vi "Read From I16 File.vi"(8 "start of read offset (bytes:0)":i32, 9 "2D number of columns/1D count (all as 1D:-1)":i32=-1, 10 "2D number of rows":i32, 11 "file path (dialog if empty)":path) -> (0 "mark after read (bytes)":i32, 1 "1D array":i16[](array[numeric]), 2 "2D array":i16[][](array[numeric]), 3 "new file path (Not A Path if cancelled)":path, 4 "EOF?":bool)   [LabVIEW 2009]
doc: "Reads a 2D or 1D array of data from a byte stream file of 16-bit signed integers."
panel:
  in  "prompt":string="Choose file to read."
  in  "instructions":string="* To read the entire file into 1D array, set 1D count <0 (default); you can leave 2D number of rows unwired.\n* To read N elements into 1D array, set 1D count =N and leave 2D number of rows wired or set to 0.\n* To read the entire file into 2D array, set 2D number of rows <0 and 2D number of columns =N >0.  The VI calculates the number of rows as the integer part of file size/N.\n* To read M rows and N columns into 2D array, set 2D number of rows =M and 2D number of columns =N."
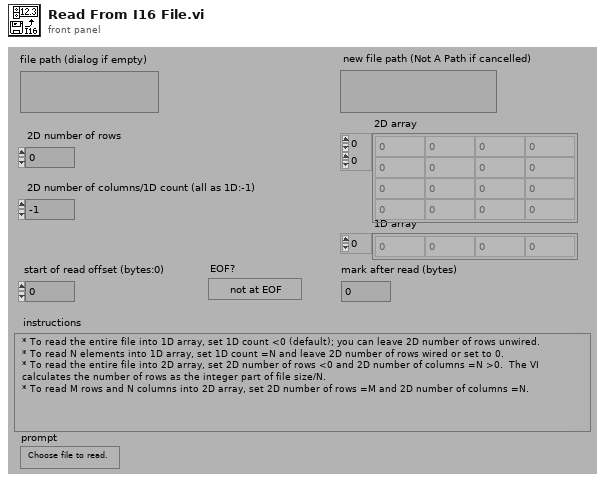
[diagram p1: front panel]
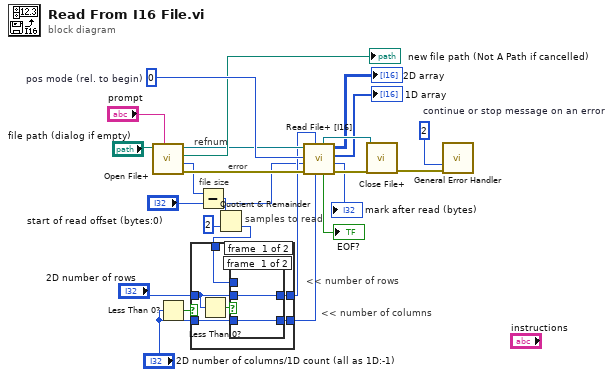
[diagram p0: block diagram]
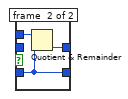
[diagram p2: hidden frame]
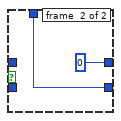
[diagram p3: hidden frame]
diagram:
  w21 = i16 0  # pos mode (rel. to begin)
  w22 = u16 2  # continue or stop message on an error
  # "samples to read"
  # "<< number of rows"
  # "<< number of columns"
  # "file size"
  # "error"
  # "refnum"
  n1 = call <vilib>:"Open File+.vi"("prompt"="prompt", "file path (\" \")"="file path (dialog if empty)") -> ("error out"=w23:errorcluster, "file size (bytes)"=w2:i32, "file path"=→"new file path (Not A Path if cancelled)":path, "refnum"=w12:refnum<file>)  [unwired: 6 in]
  n2 = Less Than 0?(x="2D number of columns/1D count (all as 1D:-1)") -> (x < 0?=w11:bool)
  n3 = Subtract(x=w2, y="start of read offset (bytes:0)") -> (x-y=w6:i32)
  n4 = Quotient & Remainder(x=w6, y=2) -> (floor(x/y)=w3:i32)  [unwired: 1 out]
  n5 = case shown="False" w11 {
    tunnel: [w29 0] -> w10
    tunnel: [w27 w36] -> w9
    tunnel: "2D number of columns/1D count (all as 1D:-1)" -> [w28 _]
    tunnel: "2D number of rows" -> [w25 _]
    tunnel: w3 -> [w26 w36]
    frame #0 {
      n6 = Less Than 0?(x=w25) -> (x < 0?=w30:bool)
      n7 = case shown="True" w30 {
        tunnel: [w31 w35] -> w29
        tunnel: w26 -> [_ w34]
        tunnel: w28 -> [w32 w33]
        tunnel: [w32 w33] -> w27
        tunnel: w25 -> [w31 _]
        frame #0 {
        }
        frame #1 {
          n8 = Quotient & Remainder(x=w34, y=w33) -> (floor(x/y)=w35:i32)  [unwired: 1 out]
        }
      }
    }
    frame #1 {
    }
  }
  n9 = call "Read File+ [I16].vi"("2D number of columns/1D count"=w9, "2D number of rows"=w10, "error in (no error)"=w23, "pos offset (bytes:0)"="start of read offset (bytes:0)", "pos mode (rel. to current:2)"=w21, "refnum"=w12) -> ("error out"=w20:errorcluster, "mark after read (bytes)"=→"mark after read (bytes)":i32, "1D data"=→"1D array":i16[], "2D data"=→"2D array":i16[][], "EOF?"=→"EOF?":bool, "dup refnum"=w16:refnum<file>)
  n10 = call <vilib>:"Close File+.vi"("error in (no error)"=w20, "refnum"=w16) -> ("error out"=w18:errorcluster)  [unwired: 3 in, 2 out]
  n11 = call <vilib>:"General Error Handler.vi"("type of dialog (OK msg:1)"=w22, "error in (no error)"=w18) -> ()  [unwired: 9 in, 5 out]
